vi "localkilenc.vi"() -> ()   [LabVIEW 2011]
panel:
  out "String":string
  out "count 2":i32
  out "count1":i32
  in  "stop":bool
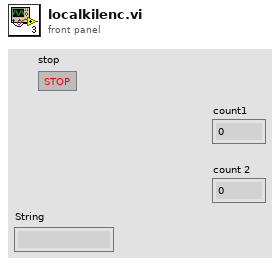
[diagram p1: front panel]
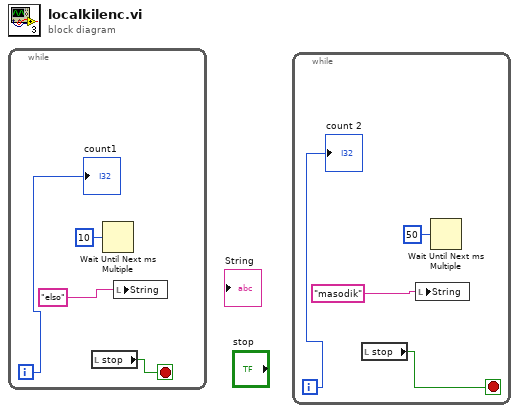
[diagram p0: block diagram]
diagram:
  n1 = while {
    i -> [w2]
    stop <- w1 stop-if-true
    n2 = local read "stop"() -> (w1:bool)
    n3 = Wait Until Next ms Multiple(millisecond multiple=u32 10) -> ()  [unwired: 1 out]
    n4 = local write "String"("elso") -> ()
    "count1" <- w2
  }
  n5 = while {
    i -> [w6]
    stop <- w5 stop-if-true
    n6 = local read "stop"() -> (w5:bool)
    n7 = local write "String"("masodik") -> ()
    n8 = Wait Until Next ms Multiple(millisecond multiple=u32 50) -> ()  [unwired: 1 out]
    "count 2" <- w6
  }
